vi "prepend time to sonde data array.vi"(9 "Measurement Labels":string[](array[string]), 10 "Sonde\nData Array":dbl[][](array[numeric]), 11 "Time Array":dbl[](array[numeric])) -> (2 "Header Array":string[](array[string]), 3 "Data Array":dbl[][](array[numeric]))   [LabVIEW 2016]
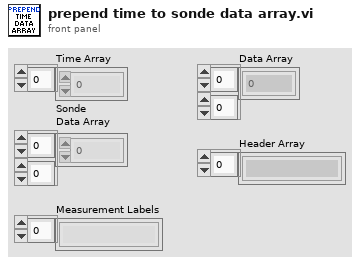
[diagram p1: front panel]
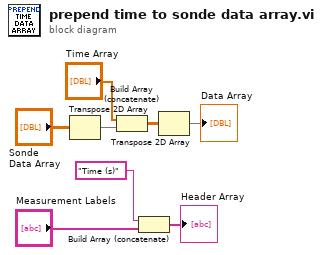
[diagram p0: block diagram]
diagram:
  n1 = Transpose 2D Array(2D array="Sonde\nData Array") -> (transposed array=w3:dbl[][])
  n2 = Build Array (concatenate)("Time Array", w3) -> (w4:dbl[][])
  n3 = Build Array (concatenate)("Time (s)", "Measurement Labels") -> (→"Header Array":string[])
  n4 = Transpose 2D Array(2D array=w4) -> (transposed array=→"Data Array":dbl[][])
